vi "Lab06.vi"() -> ()   [LabVIEW 2022 SP3]
uses:
  <vilib>/measure/NI_MABase.lvlib
panel:
  in  "STOP":bool
  out "Sine Wave":waveform(dbl)(graph)
  in  "Amplitude":dbl(knob) scale=0.0..10.0
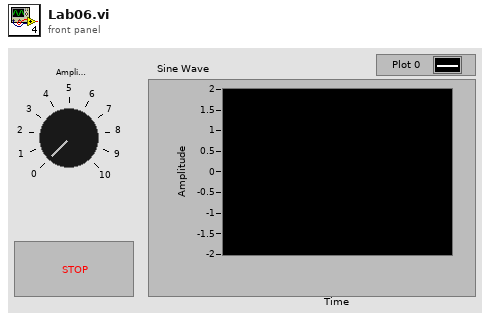
[diagram p1: front panel]
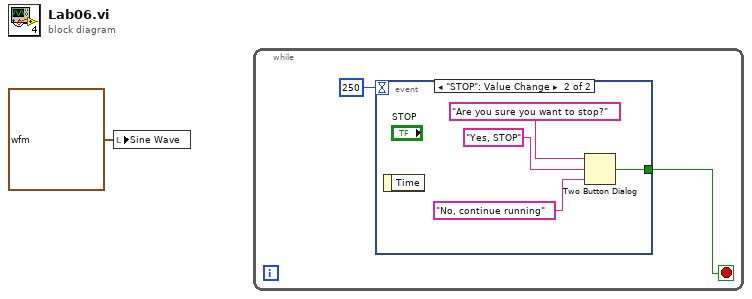
[diagram p0: block diagram]
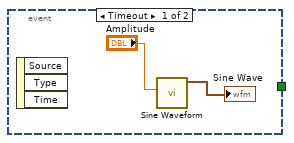
[diagram p2: hidden frame]
diagram:
  n1 = local write "Sine Wave"(waveform(dbl) {"t0"=timestamp(0 s since 1904-01-01), "dt"=0.0, "Y"=[]} ("Sine Wave")) -> ()
  n2 = while {
    stop <- w2 stop-if-true
    n3 = event shown="[1] \"STOP\": Value Change" {
      selector: _ -> [_ _]
      dyn-events: _ -> [_ _]
      timeout: 250 -> [_ _]
      tunnel: [_ w6] -> w2
      event Timeout {
        n4 = event-data() -> ()  [unwired: 1 in, 3 out]
        n5 = call <vilib>:"Sine Waveform.vi"("amplitude"="Amplitude") -> ("signal out"=→"Sine Wave":waveform(dbl))  [unwired: 9 in, 1 out]
      }
      event "STOP": Value Change {
        n6 = event-data() -> ()  [unwired: 1 in, 1 out]
        n7 = Two Button Dialog(message="Are you sure you want to stop?", 1:"No, continue running" ("Center Button Text (\"No\")"), 2:"Yes, STOP" ("Left Button Text (\"Yes\")")) -> (T button?=w6:bool)
      }
    }
  }
